vi "Proportional area crop.vi"(6 "Cropped to area pixels":u32=1048576, 7 "keep aspect ratio":bool=TRUE, 8 "Y grids":u8=1, 9 "Y resolution":u32, 10 "X grids":u8=1, 11 "X resolution":u32) -> (0 "Y length":u32, 1 "Y index":u32[](array[numeric]), 2 "X length":u32, 3 "X index":u32[](array[numeric]))   [LabVIEW 2018]
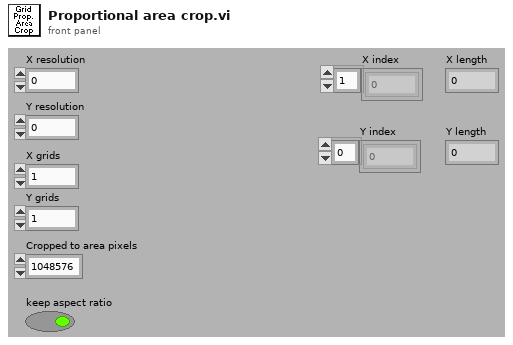
[diagram p1: front panel]
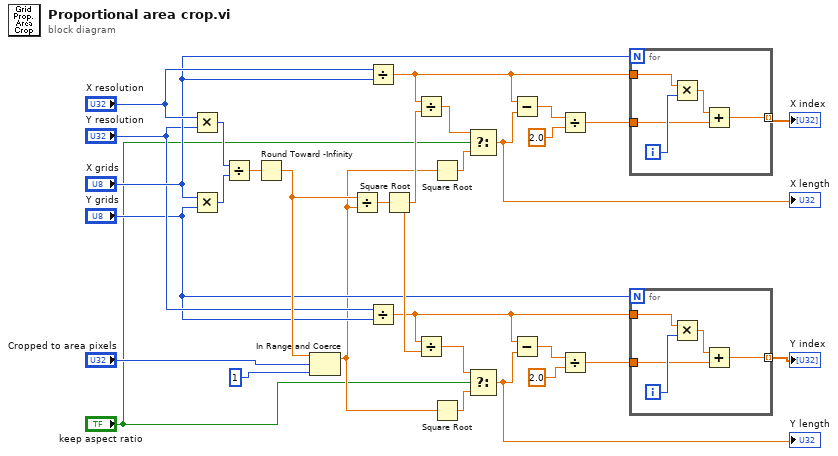
[diagram p0: block diagram]
diagram:
  n1 = Multiply(x="X resolution", y="Y resolution") -> (x*y=w20:u32)
  n2 = Multiply(x="X grids", y="Y grids") -> (x*y=w22:u8)
  n3 = Divide(x=w20, y=w22) -> (x/y=w21:dbl)
  n4 = Round Toward -Infinity(1:w21) -> (0:w15:dbl)
  n5 = In Range and Coerce(upper limit=w15, x="Cropped to area pixels", lower limit=u32 1) -> (coerced(x)=w3:dbl)  [unwired: 1 out]
  n6 = Divide(x=w15, y=w3) -> (x/y=w26:dbl)
  n7 = Divide(x="X resolution", y="X grids") -> (x/y=w10:dbl)
  n8 = Divide(x="Y resolution", y="Y grids") -> (x/y=w9:dbl)
  n9 = Square Root(x=w26) -> (sqrt(x)=w25:dbl)
  n10 = Divide(x=w10, y=w25) -> (x/y=w8:dbl)
  n11 = Divide(x=w9, y=w25) -> (x/y=w4:dbl)
  n12 = Square Root(x=w3) -> (sqrt(x)=w6:dbl)
  n13 = Square Root(x=w3) -> (sqrt(x)=w5:dbl)
  n14 = Select(t=w8, s="keep aspect ratio", f=w6) -> (s? t:f=w7:dbl)
  "X length" <- w7
  n15 = Select(t=w4, s="keep aspect ratio", f=w5) -> (s? t:f=w1:dbl)
  "Y length" <- w1
  n16 = Subtract(x=w10, y=w7) -> (x-y=w27:dbl)
  n17 = Subtract(x=w9, y=w1) -> (x-y=w30:dbl)
  n18 = Divide(x=w27, y=2.0) -> (x/y=w19:dbl)
  n19 = Divide(x=w30, y=2.0) -> (x/y=w17:dbl)
  n20 = for {
    N: "X grids" -> [_]
    tunnel: w19 -> [w32]
    tunnel: w10 -> [w34]
    tunnel: [w31] -> w18 mode=indexing
    i -> [w35]
    n21 = Multiply(x=w34, y=w35) -> (x*y=w33:dbl)
    n22 = Add(x=w33, y=w32) -> (x+y=w31:dbl)
  }
  "X index" <- w18
  n23 = for {
    N: "Y grids" -> [_]
    tunnel: w17 -> [w37]
    tunnel: w9 -> [w39]
    tunnel: [w36] -> w16 mode=indexing
    i -> [w40]
    n24 = Multiply(x=w39, y=w40) -> (x*y=w38:dbl)
    n25 = Add(x=w38, y=w37) -> (x+y=w36:dbl)
  }
  "Y index" <- w16
